vi "filepath_from_path.vi"(8 "error in (no error)":errorcluster, 10 "path":string, 11 "filepath in":path) -> (0 "error out":errorcluster, 3 "filepath out":path)   [LabVIEW 2015, in "lv-dropbox.lvlib"]
uses:
  lv-dropbox.lvlib
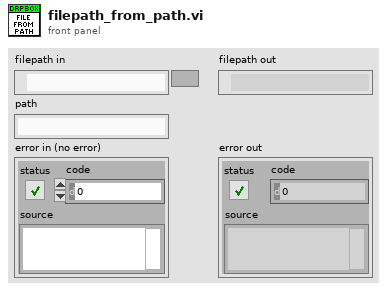
[diagram p1: front panel]
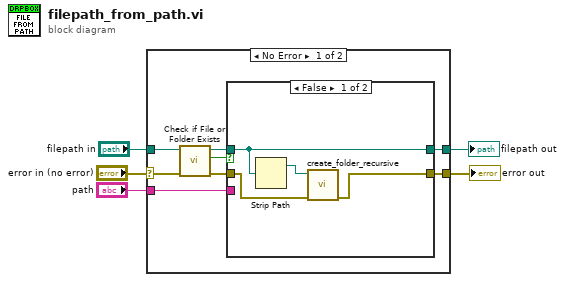
[diagram p0: block diagram]
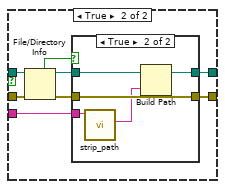
[diagram p2: hidden frame]
diagram:
  n1 = case shown="No Error" "error in (no error)" {
    selector: "error in (no error)" -> [w10 w34]
    tunnel: "filepath in" -> [w11 w33]
    tunnel: "path" -> [w13 _]
    tunnel: [w7 w33] -> w2
    tunnel: [w12 w34] -> w1
    frame No Error {
      n2 = call <vilib>:"Check if File or Folder Exists.vi"("error in (no error)"=w10, "path"=w11) -> ("error out"=w9:errorcluster, "file or folder exists?"=w6:bool, "dup path"=w8:path)  [unwired: 7 in]
      n3 = case shown="False" w6 {
        tunnel: w13 -> [_ w25]
        tunnel: [w15 w21] -> w12
        tunnel: w9 -> [w17 w20]
        tunnel: w8 -> [w14 w19]
        tunnel: [w14 w18] -> w7
        frame False {
          n4 = Strip Path(path=w14) -> (stripped path=w16:path)  [unwired: 1 out]
          n5 = call "create_folder_recursive.vi"("error in"=w17, "path in"=w16) -> ("error out"=w15:errorcluster)  [unwired: 8 in, 1 out]
        }
        frame True {
          n6 = File/Directory Info(path=w19, error in=w20) -> (path out=w22:path, directory=w24:bool, error out=w23:errorcluster)  [unwired: 4 out]
          n7 = case shown="True" w24 {
            tunnel: w25 -> [_ w30]
            tunnel: w23 -> [w26 w29]
            tunnel: w22 -> [w27 w32]
            tunnel: [w27 w31] -> w18
            tunnel: [w26 w29] -> w21
            frame False {
            }
            frame True {
              n8 = call "strip_path.vi"("path"=w30) -> ("name"=w28:string)  [unwired: 9 in, 1 out]
              n9 = Build Path(base path=w32, name or relative path=w28) -> (appended path=w31:path)
            }
          }
        }
      }
    }
    frame Error {
    }
  }
  "error out" <- w1
  "filepath out" <- w2
